vi "LDCT.vi"(8 "error in (no error)":errorcluster, 11 "Debug":bool) -> (0 "error out":errorcluster, 3 "DeviceNum":i32)   [LabVIEW 2020, in "LDCT.lvlib"]
uses:
  LDCT.lvlib
  SQLiteBase.lvlib
  LabSCADACommon.lvlib
  Driver/DriverCommon.lvlib
  CCTM.lvlib
  Logger.lvlib
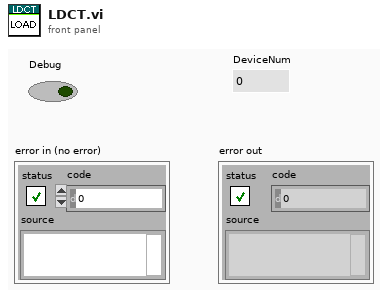
[diagram p1: front panel]
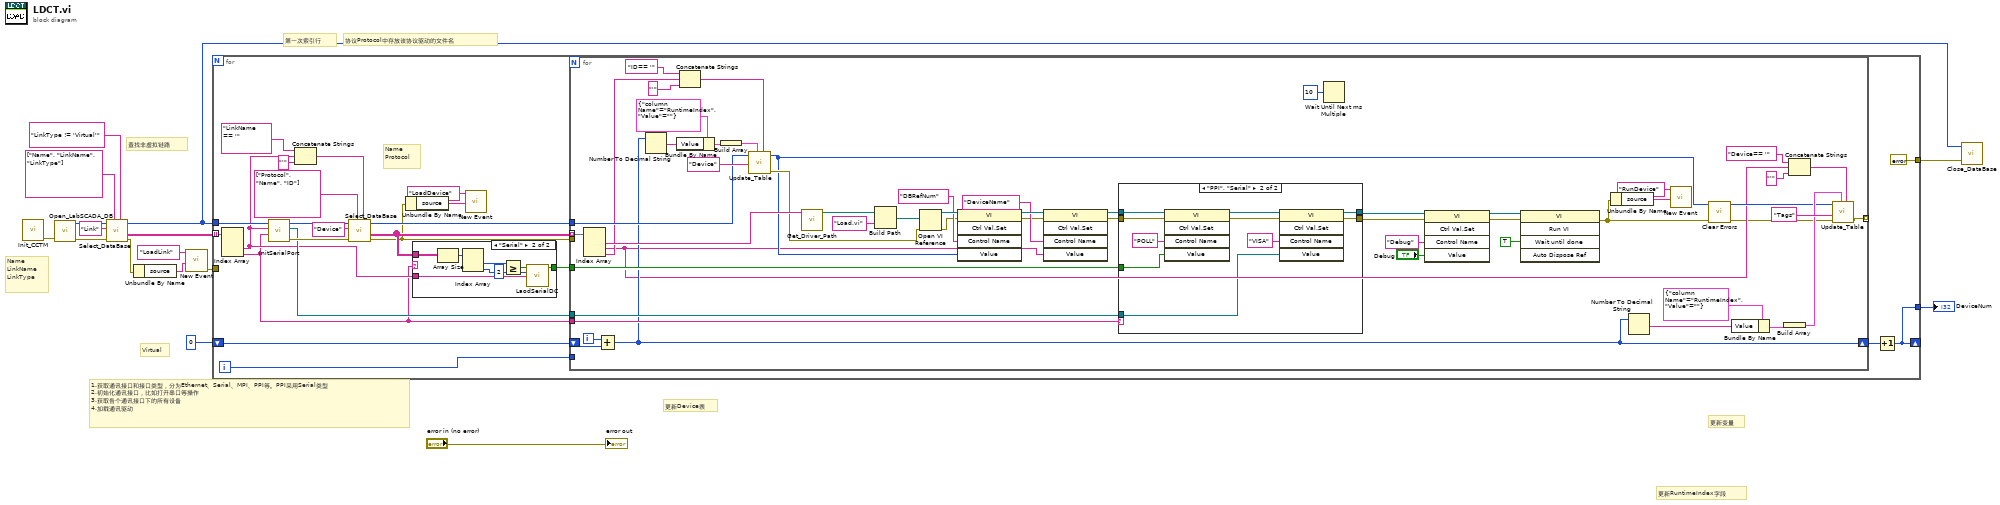
[diagram p0: block diagram]
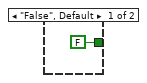
[diagram p2: hidden frame]
diagram:
  # "更新变量"
  # "更新Device表"
  # "更新RuntimeIndex字段"
  # "Virtual"
  # "Name\nLinkName\nLinkType"
  # "查找非虚拟链路"
  # "协议Protocol中存放该协议驱动的文件名"
  # "第一次索引行"
  # "1.获取通讯接口和接口类型，分为Ethernet、Serial、MPI、PPI等。PPI采用Serial类型\n2.初始化通讯接口，比如打开串口等操作\n3.获取各个通讯接口下的所有设备\n4.加载通讯驱动"
  n1 = call "Init_CCTM.vi"() -> ("error out"=w15:errorcluster)  [unwired: 11 in]
  n2 = call "Open_LabSCADA_DB.vi"("error in (no error)"=w15) -> ("error out"=w11:errorcluster, "DB Reference Out"=w10:i32)  [unwired: 9 in]
  n3 = call "Select_DataBase.vi"("Expression"="LinkType != 'Virtual'", "Query Columns"=string[] ["Name", "LinkName", "LinkType"], "error in (no error)"=w11, "Table name"="Link", "DB Reference In"=w10) -> ("error out"=w5:errorcluster, "Data"=w9:string[][], "DB Reference Out"=w8:i32)  [unwired: 4 in]
  n4 = Unbundle By Name(w5) -> ("source"=w4:string)
  n5 = call "New Event.vi"("Information"=w4, "Event"="LoadLink") -> ("error out"=w3:errorcluster)  [unwired: 8 in, 1 out]
  n6 = for {
    tunnel: w9 -> [w35] mode=indexing
    tunnel: w8 -> [w31]
    tunnel: [errorcluster {"status"=FALSE, "code"=0, "source"=""} ("error constant")] -> w7
    tunnel: w3 -> [_]
    shift-right: [w17] -> _
    shift-left: 0 -> [w19]
    tunnel: [w17] -> w1
    i -> [w20]
    # "Name\nProtocol"
    n7 = Index Array(array=w35) -> (element #2=w26:string, element #3=w24:string)  [unwired: 3 in, 1 out]
    n8 = call "InitSerialPort.vi"("LinkType"=w24, "LinkName"=w26, "DBRefNum"=w31) -> ("error out"=w29:errorcluster, "VISA resource name out"=w28:refnum<visa-resource-name>, "DB Reference Out"=w30:i32)  [unwired: 6 in]
    n9 = Concatenate Strings("LinkName == '" ("Expression"), w26, "'" ("string")) -> (w33:string)
    n10 = call "Select_DataBase.vi"("Expression"=w33, "Query Columns"=string[] ["Protocol", "Name", "ID"], "error in (no error)"=w29, "Table name"="Device", "DB Reference In"=w30) -> ("error out"=w23:errorcluster, "Data"=w32:string[][], "DB Reference Out"=w36:i32)  [unwired: 4 in]
    n11 = Unbundle By Name(w23) -> ("source"=w22:string)
    n12 = case shown="\"Serial\"" w24 {
      tunnel: w32 -> [_ w48]
      tunnel: [FALSE ("POLL?") w43] -> w27
      tunnel: w26 -> [_ w41]
      frame "False", Default {
      }
      frame "Serial" {
        n13 = Array Size(array=w48) -> (size(s)=w47:i32[])
        n14 = Index Array(array=w47) -> (element #1=w46:i32, element #2=w42:i32)  [unwired: 2 in]
        n15 = Greater Or Equal?(x=w46, y=2) -> (x >= y?=w44:bool)
        n16 = call "LaodSerialDC.vi"("Interface"=w41, "DeviceQuantity"=w42, "POLL"=w44) -> ("POLL?"=w43:bool)  [unwired: 7 in, 1 out]
      }
    }
    n17 = call "New Event.vi"("Information"=w22, "Event"="LoadDevice") -> ()  [unwired: 8 in, 2 out]
    n18 = for {
      tunnel: w32 -> [w101] mode=indexing
      tunnel: w36 -> [w58]
      tunnel: w23 -> [_]
      tunnel: w24 -> [w89]
      tunnel: w27 -> [w87]
      tunnel: w28 -> [w88]
      tunnel: w20 -> [_]
      tunnel: [w76] -> _ mode=indexing
      shift-right: [w56] -> w18
      shift-left: w19 -> [w74]
      i -> [w75]
      n19 = Index Array(array=w101) -> (element #1=w90:string, element #2=w54:string, element #3=w57:string)  [unwired: 3 in]
      n20 = Add(x=w75, y=w74) -> (x+y=w56:i32)
      n21 = Number To Decimal String(number=w56) -> (decimal integer string=w67:string)  [unwired: 1 in]
      n22 = Bundle By Name(cluster=cluster{"column Name":string, "Value":string} {"column Name"="RuntimeIndex", "Value"=""} ("cell"), "Value"=w67) -> (w65:cluster{"column Name":string, "Value":string})
      n23 = Concatenate Strings("ID== '" ("Expression"), w57, "'" ("string")) -> (w64:string)
      n24 = Build Array(w65) -> (w66:cluster{"column Name":string, "Value":string}[])
      n25 = call "Update_Table.vi"("Expression"=w64, "Columns"=w66, "Table Name"="Device", "DB Reference In"=w58) -> ("error out"=w59:errorcluster, "DB Reference Out"=w55:i32)  [unwired: 6 in]
      n26 = call "Get_Driver_Path.vi"("Driver Filename"=w90) -> ("Driver Path"=w94:path)  [unwired: 10 in]
      n27 = Build Path(base path=w94, name or relative path="Load.vi") -> (appended path=w93:path)
      n28 = Open VI Reference(vi path=w93, error in (no error)=w59) -> (vi reference=w99:refnum<vi>, error out=w92:errorcluster)  [unwired: 4 in]
      n29 = invoke class="VI" method="Ctrl Val.Set"(reference=w99, error in=w92, "Control Name"="DBRefNum", "Value"=w55) -> (reference out=w97:refnum<vi>, error out=w91:errorcluster)  [unwired: 1 in, 3 out]
      n30 = invoke class="VI" method="Ctrl Val.Set"(reference=w97, error in=w91, "Control Name"="DeviceName", "Value"=w54) -> (reference out=w86:refnum<vi>, error out=w85:errorcluster)  [unwired: 1 in, 3 out]
      n31 = case shown="\"PPI\", \"Serial\"" w89 {
        tunnel: [w103 w112] -> w73
        tunnel: w86 -> [w103 w105]
        tunnel: [w102 w113] -> w72
        tunnel: w85 -> [w102 w104]
        tunnel: w88 -> [_ w110]
        tunnel: w87 -> [_ w108]
        frame "False", Default {
        }
        frame "PPI", "Serial" {
          n32 = invoke class="VI" method="Ctrl Val.Set"(reference=w105, error in=w104, "Control Name"="POLL", "Value"=w108) -> (reference out=w107:refnum<vi>, error out=w106:errorcluster)  [unwired: 1 in, 3 out]
          n33 = invoke class="VI" method="Ctrl Val.Set"(reference=w107, error in=w106, "Control Name"="VISA", "Value"=w110) -> (reference out=w112:refnum<vi>, error out=w113:errorcluster)  [unwired: 1 in, 3 out]
        }
      }
      n34 = Wait Until Next ms Multiple(millisecond multiple=u32 10) -> ()  [unwired: 1 out]
      n35 = invoke class="VI" method="Ctrl Val.Set"(reference=w73, error in=w72, "Control Name"="Debug", "Value"="Debug") -> (reference out=w71:refnum<vi>, error out=w70:errorcluster)  [unwired: 1 in, 3 out]
      n36 = invoke class="VI" method="Run VI"(reference=w71, error in=w70, "Wait until done"=TRUE ("Wait Until Done")) -> (error out=w51:errorcluster)  [unwired: 2 in, 4 out]
      n37 = Unbundle By Name(w51) -> ("source"=w53:string)
      n38 = Number To Decimal String(number=w56) -> (decimal integer string=w77:string)  [unwired: 1 in]
      n39 = call "New Event.vi"("Information"=w53, "Event"="RunDevice") -> ()  [unwired: 8 in, 2 out]
      n40 = call <vilib>:"Clear Errors.vi"("error in (no error)"=w51) -> ("error out"=w50:errorcluster)  [unwired: 5 in, 1 out]
      n41 = Bundle By Name(cluster=cluster{"column Name":string, "Value":string} {"column Name"="RuntimeIndex", "Value"=""} ("cell"), "Value"=w77) -> (w79:cluster{"column Name":string, "Value":string})
      n42 = Build Array(w79) -> (w78:cluster{"column Name":string, "Value":string}[])
      n43 = Concatenate Strings("Device== '" ("Expression"), w54, "'" ("string")) -> (w81:string)
      n44 = call "Update_Table.vi"("Expression"=w81, "Columns"=w78, "error in (no error)"=w50, "Table Name"="Tags", "DB Reference In"=w55) -> ("error out"=w76:errorcluster)  [unwired: 5 in, 1 out]
    }
    n45 = Increment(x=w18) -> (x+1=w17:i32)
  }
  "DeviceNum" <- w1
  n46 = call "Close_DataBase.vi"("error in (no error)"=w7, "DB Reference In"=w8) -> ()  [unwired: 9 in, 1 out]
  "error out" <- "error in (no error)"
